vi "frontp_get_subpanel_reference.vi"(8 "error in (no error)":errorcluster, 10 "hardware":T1, 11 "front_panel in":refnum<class "front_panel.lvclass">) -> (0 "error out":errorcluster, 2 "subpanel":refnum<vi>, 3 "front_panel out":refnum<class "front_panel.lvclass">)   [LabVIEW 2015, in "front_panel.lvclass"]
uses:
  front_panel.lvclass
  hardware_caller_queue_numbers.ctl
  front_panel.lvclass/front_panel.ctl
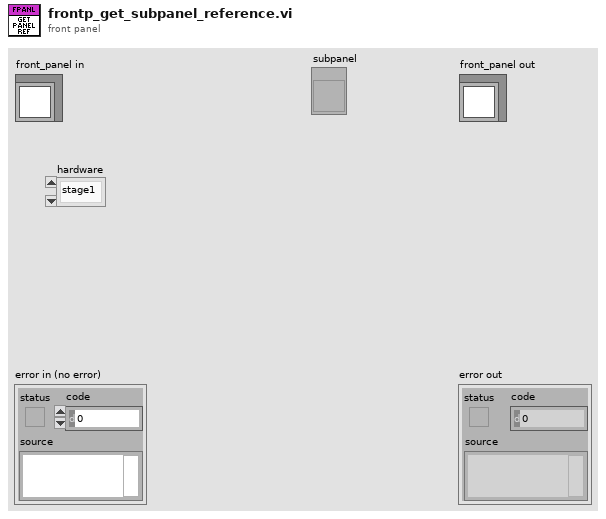
[diagram p1: front panel]
types:
  T1 = typedef "hardware_caller_queue_numbers.ctl" = enum16{"stage1", "stage2", "experiment", "detector"}
  T2 = typedef "gui_subpanel_references.ctl" = cluster{"Stage 1":refnum<vi>, "Stage 2":refnum<vi>, "Experiment":refnum<vi>, "Detector":refnum<vi>}
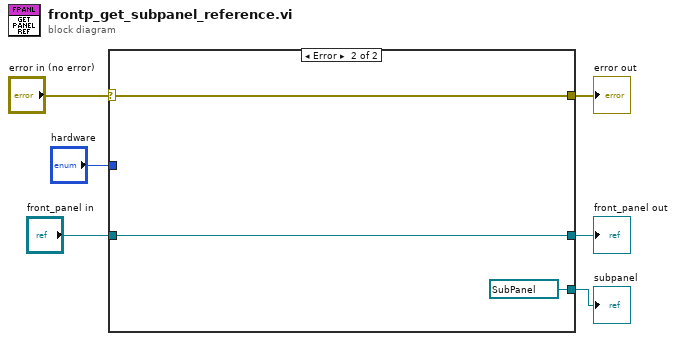
[diagram p0: block diagram]
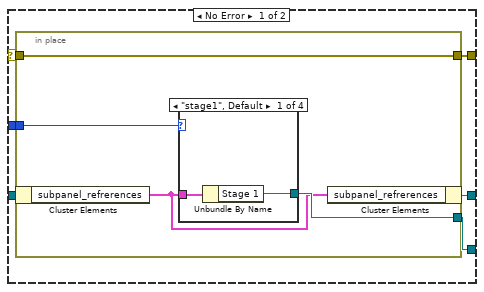
[diagram p2: hidden frame]
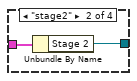
[diagram p3: hidden frame]
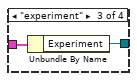
[diagram p4: hidden frame]
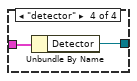
[diagram p5: hidden frame]
diagram:
  n1 = case shown="Error" "error in (no error)" {
    selector: "error in (no error)" -> [w11 w27]
    tunnel: [w7 w27] -> w5
    tunnel: [w9 w26] -> w3
    tunnel: "front_panel in" -> [w12 w26]
    tunnel: "hardware" -> [w10 _]
    tunnel: [w8 refnum<vi> refnum ("Detector")] -> w1
    frame No Error {
      n2 = in-place {
        in-place-border: w11 -> [w14]
        in-place-border: w10 -> [w16]
        in-place-border: [w15] -> w8
        in-place-border: [w14] -> w7
        n3 = in-place-cluster #1(w12) -> ("subpanel_refrerences"=w13:T2)
        n4 = case shown="\"stage1\", Default" w16 {
          tunnel: w13 -> [w18 w20 w22 w24]
          tunnel: [w17 w19 w21 w23] -> w15
          frame "stage1", Default {
            n5 = Unbundle By Name(w18) -> ("Stage 1"=w17:refnum<vi>)
          }
          frame "stage2" {
            n6 = Unbundle By Name(w20) -> ("Stage 2"=w19:refnum<vi>)
          }
          frame "experiment" {
            n7 = Unbundle By Name(w22) -> ("Experiment"=w21:refnum<vi>)
          }
          frame "detector" {
            n8 = Unbundle By Name(w24) -> ("Detector"=w23:refnum<vi>)
          }
        }
        n9 = in-place-cluster #1("subpanel_refrerences"=w13) -> (w9:refnum<class "front_panel.lvclass">)
      }
    }
    frame Error {
    }
  }
  "error out" <- w5
  "front_panel out" <- w3
  "subpanel" <- w1
